vi "Build State URL.vi"(9 "ID":u8, 10 "Hue Config":T1) -> (2 "URL":string)   [LabVIEW 2020, in "LMH-Hue.lvlib"]
uses:
  LMH-Hue.lvlib
  Type Defs/Hue Ref.ctl
  <vilib>/httpClient/ClientHandle.ctl
  Type Defs/Light Data.ctl
  <vilib>/httpClient/LabVIEWHTTPClient.lvlib
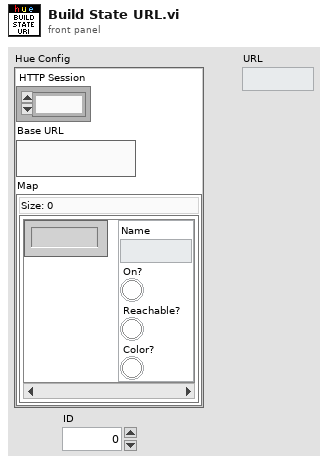
[diagram p1: front panel]
types:
  T1 = typedef "LMH-Hue.lvlib/Hue Ref.ctl" = cluster{"HTTP Session":T2, "Base URL":string, "Map":map{i32, T3}}
  T2 = typedef "LabVIEWHTTPClient.lvlib/ClientHandle.ctl" = refnum<k1>
  T3 = typedef "LMH-Hue.lvlib/Light Data.ctl" = cluster{"Name":string, "On?":bool, "Reachable?":bool, "Color?":bool}
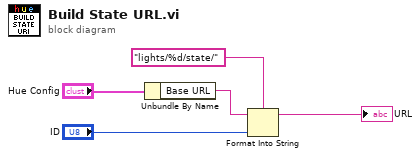
[diagram p0: block diagram]
diagram:
  n1 = Unbundle By Name("Hue Config") -> ("Base URL"=w1:string)
  n2 = Format Into String(format string="lights/%d/state/", initial string=w1, "ID") -> (resulting string=→"URL":string)  [unwired: 1 in, 1 out]
